vi "Write FGV Data.vi"(0 "AI in":refnum<class "AI.lvclass">, 1 "0Cv/1St":i32, 5 "DataIn":string, 7 "Data":T1=enum."CurrentAction", 11 "error in (no error)":errorcluster) -> (4 "AI out":refnum<class "AI.lvclass">, 15 "error out":errorcluster)   [LabVIEW 2019, in "AI.lvclass"]
uses:
  AI.lvclass
  Ctrl/Auto Inspection Data Name.ctl
  Ctrl/Auto Inspection Station Name2.ctl
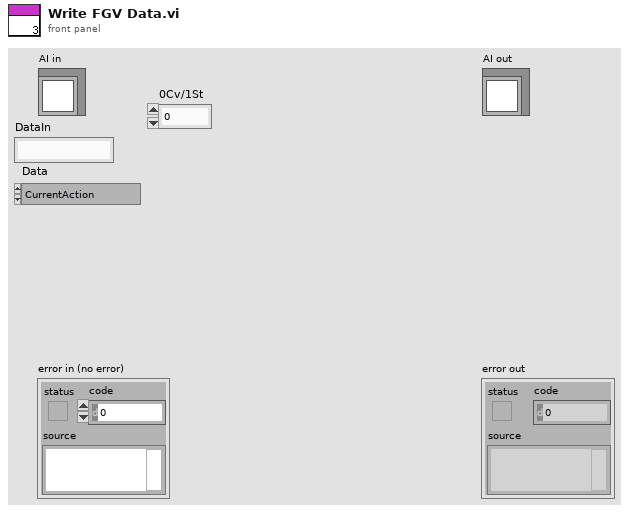
[diagram p1: front panel]
types:
  T1 = typedef "Auto Inspection Data Name.ctl" = enum16{"LocalRun", "ItemSN(TimeCode)", "CurrentAction", "Error", "Data", "OKNG", "電壓值", "電壓值判斷", "電流值", "電流值判斷", "Laser1 Data", "Laser2 Data", "Laser OKNG", "StationNO"}
  T2 = typedef "Auto Inspection Station Name2.ctl" = enum16{"S1Barcode", "S2Measure", "S3Measure", "S4Measure", "S5Measure", "S11_LaserCheck", "S8_Vision AI"}
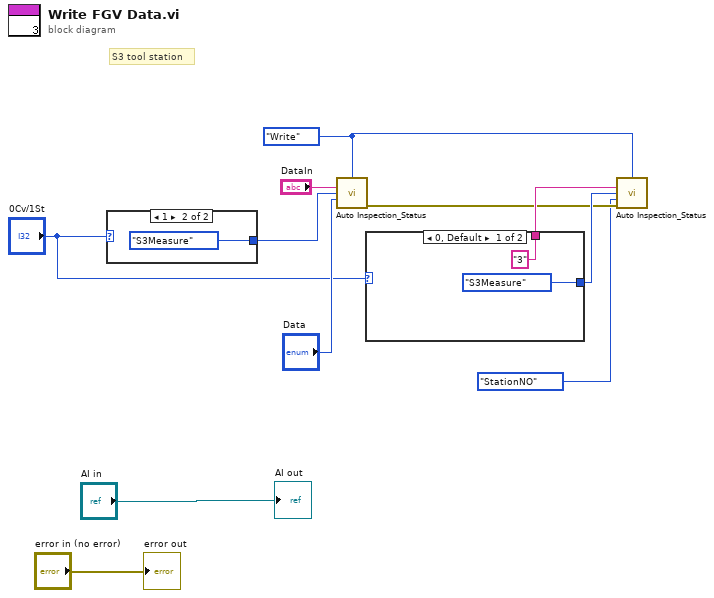
[diagram p0: block diagram]
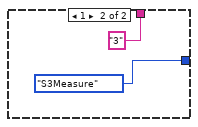
[diagram p2: hidden frame]
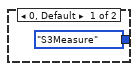
[diagram p3: hidden frame]
diagram:
  w6 = enum16{"Initial", "Write", "Read"}."Write" ("Action")
  # "S3 tool station"
  n1 = case shown="1" "0Cv/1St" {
    tunnel: [Auto_Inspection_Station_Name2."S3Measure" ("Station") Auto_Inspection_Station_Name2."S3Measure" ("Station")] -> w11
    frame 0, Default {
    }
    frame 1 {
    }
  }
  n2 = call "Auto Inspection_Status.vi"("Action"=w6, "DataIn"="DataIn", "Station"=w11, "Data"="Data") -> ("error out"=w2:errorcluster)  [unwired: 9 in, 2 out]
  n3 = case shown="0, Default" "0Cv/1St" {
    tunnel: [Auto_Inspection_Station_Name2."S3Measure" ("Station") Auto_Inspection_Station_Name2."S3Measure" ("Station")] -> w5
    tunnel: ["3" "3"] -> w3
    frame 0, Default {
    }
    frame 1 {
    }
  }
  n4 = call "Auto Inspection_Status.vi"("Action"=w6, "DataIn"=w3, "Station"=w5, "Data"=Auto_Inspection_Data_Name."StationNO", "error in"=w2) -> ()  [unwired: 8 in, 3 out]
  "error out" <- "error in (no error)"
  "AI out" <- "AI in"
